vi "my_daq_audio.vi"() -> ()   [LabVIEW 2018]
panel:
  in  "volume":dbl(knob) scale=0.0..1.0
  in  "treble":dbl(knob) scale=0.0..2.0
  in  "mid":dbl(knob) scale=0.0..2.0
  in  "bass":dbl(knob) scale=0.0..2.0
  in  "stop":bool
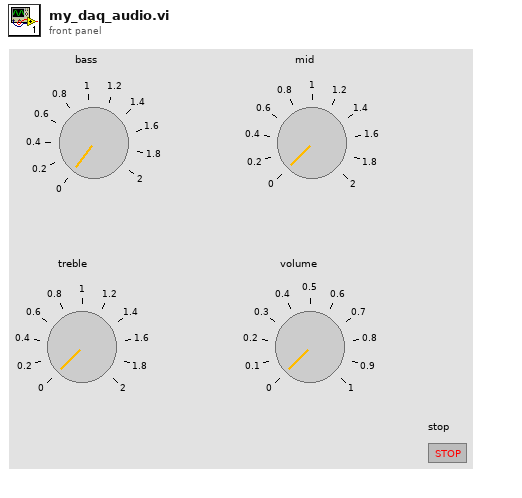
[diagram p1: front panel]
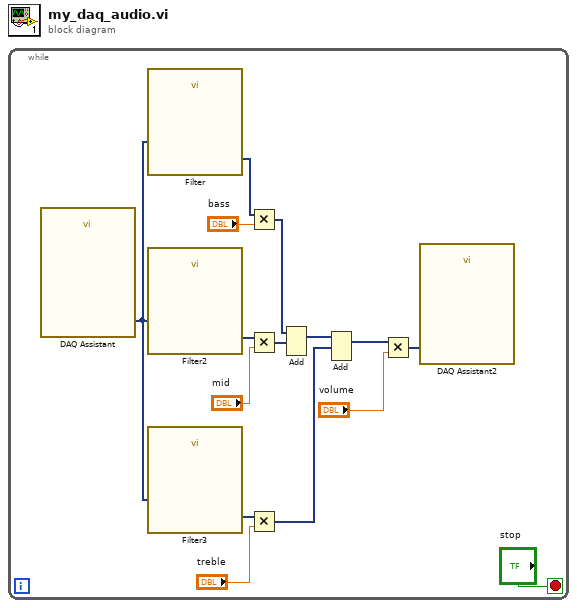
[diagram p0: block diagram]
diagram:
  n1 = while {
    stop <- "stop" stop-if-true
    n2 = call "DAQ Assistant"() -> ("data"=w14:dynamicdata)  [unwired: 16 in, 3 out]
    n3 = call "Filter"("Signal"=w14) -> ("Filtered Signal"=w12:dynamicdata)  [unwired: 9 in, 1 out]
    n4 = call "Filter2"("Signal"=w14) -> ("Filtered Signal"=w10:dynamicdata)  [unwired: 9 in, 1 out]
    n5 = call "Filter3"("Signal"=w14) -> ("Filtered Signal"=w9:dynamicdata)  [unwired: 9 in, 1 out]
    n6 = Multiply(x=w12, y="bass") -> (x*y=w7:dynamicdata)
    n7 = Multiply(x=w10, y="mid") -> (x*y=w6:dynamicdata)
    n8 = Multiply(x=w9, y="treble") -> (x*y=w4:dynamicdata)
    n9 = Add(1:w6, 2:w7) -> (0:w5:dynamicdata)  [unwired: 1 in, 1 out]
    n10 = Add(1:w4, 2:w5) -> (0:w3:dynamicdata)  [unwired: 1 in, 1 out]
    n11 = Multiply(x=w3, y="volume") -> (x*y=w1:dynamicdata)
    n12 = call "DAQ Assistant2"("data"=w1) -> ()  [unwired: 16 in, 3 out]
  }
